vi "Update Fan Status.vi"(8 "error in (no error)":cluster{"状态":bool, "代码":i32, "源":string} caption="错误输入（无错误）", 9 "风扇B":T1, 10 "风扇A":T1, 11 "蒸发冷却器":refnum<class "Evaporative Cooler.lvclass">) -> (0 "error out":cluster{"状态":bool, "代码":i32, "源":string} caption="错误输出", 3 "蒸发冷却器":refnum<class "Evaporative Cooler.lvclass">)   [LabVIEW 2015, in "Evaporative Cooler.lvlib" / "Evaporative Cooler.lvclass"]
doc: "该方法向控制器发送消息，通知两个风扇的相关信息。"
uses:
  Evaporative Cooler/Evaporative Cooler/Evaporative Cooler.lvclass
  Dual Fan/Dual Fan/Fan Info.ctl
  <vilib>/ActorFramework/Message Enqueuer/Message Enqueuer.lvclass
  Cooler.lvclass/Cooler.ctl
  Evaporative Cooler Controller/Update Fan Status Msg/Update Fan Status Msg.lvclass/Update Fan Status Msg.ctl
  <vilib>/ActorFramework/Message Enqueuer/Message Enqueuer.lvclass/Message Enqueuer.ctl
  <vilib>/ActorFramework/Message Enqueuer/Enqueue.vi
  <vilib>/ActorFramework/Message Priority Queue/Priority Enqueue.vi
  Evaporative Cooler Controller/Update Fan Status Msg/Update Fan Status Msg.lvclass
  Cooler.lvclass
  Dual Fan/Dual Fan/Dual Fan.lvclass
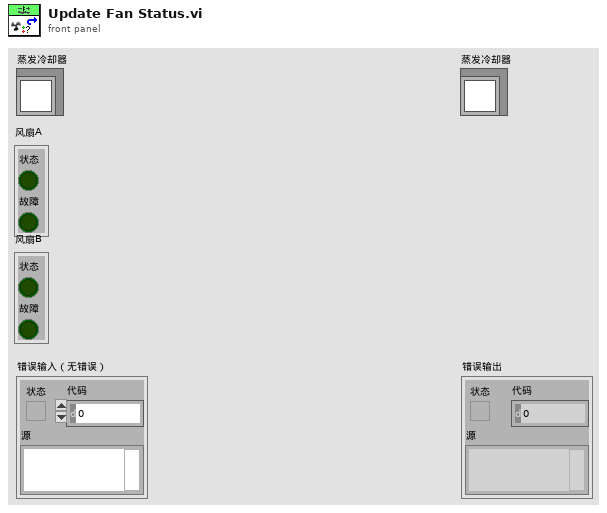
[diagram p1: front panel]
types:
  T1 = typedef "Dual Fan.lvlib/Dual Fan.lvclass/Fan Info.ctl" = cluster{"状态":bool, "故障":bool}
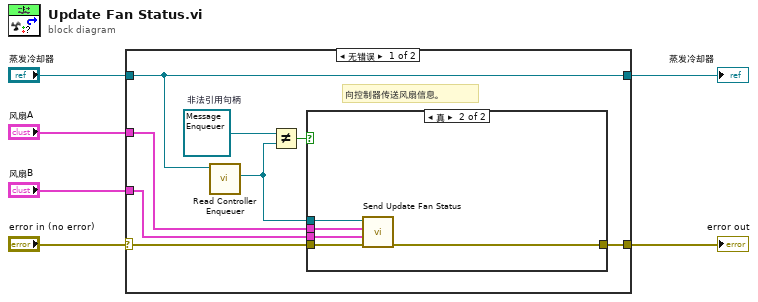
[diagram p0: block diagram]
diagram:
  n1 = case shown="无错误" "error in (no error)" {
    selector: "error in (no error)" -> [w11 w22]
    tunnel: [w10 w22] -> w5
    tunnel: [w14 w21] -> w3
    tunnel: "蒸发冷却器" -> [w14 w21]
    tunnel: "风扇A" -> [w13 _]
    tunnel: "风扇B" -> [w12 _]
    frame No Error {
      w8 = refnum<class "Message Enqueuer.lvclass"> refnum  # 非法引用句柄
      # "向控制器传送风扇信息。"
      n2 = call "Read Controller Enqueuer.vi"("冷却器"=w14) -> ("控制器待入队列"=w9:refnum<class "Message Enqueuer.lvclass">)  [unwired: 10 in]
      n3 = Not Equal?(x=w8, y=w9) -> (x != y?=w7:bool)
      n4 = case shown="真" w7 {
        tunnel: w9 -> [_ w20]
        tunnel: w13 -> [_ w19]
        tunnel: w12 -> [_ w18]
        tunnel: w11 -> [w15 w17]
        tunnel: [w15 w16] -> w10
        frame False {
        }
        frame True {
          n5 = call "Send Update Fan Status.vi"("error in (no error)"=w17, "风扇B"=w18, "风扇A"=w19, "消息待入队列"=w20) -> ("error out"=w16:cluster{"状态":bool, "代码":i32, "源":string})  [unwired: 7 in]
        }
      }
    }
    frame Error {
    }
  }
  "error out" <- w5
  "蒸发冷却器" <- w3
